vi "AlliGator All ROIs Decay Fit Non-Interactive (Fast + Individual IRF) v2.vi"(8 "error in (no error)":errorcluster, 11 "AlliGator Internal Variables DVR":refnum<data-value>) -> (0 "error out":errorcluster, 1 "Message":string, 3 "AlliGator Internal Variables DVR":refnum<data-value>)   [LabVIEW 2021, in "AlliGator Decay Analysis.lvlib" / "AlliGator Decay Fit.lvlib"]
doc: "Performs multi-ROIs NLSF decay fits for the selected ROIs.\n\nEach ROI has its own associated IRF."
uses:
  AlliGator Decay Fit.lvlib
  AlliGator Variables List.ctl
  AlliGator Globals, Variables & Constants.lvlib
  Image/Named ROI Description.ctl
  Image/Image.lvlib
  AlliGator Decay Processing.lvlib
  AlliGator Source Image.lvlib
  <vilib>/vision/Image Controls.llb/IMAQ Image.ctl
  Strings/Strings.lvlib
  Time/Time.lvlib
  AlliGator Settings.lvlib
  AlliGator Settings List.ctl
  AlliGator Abort.vi
  Variant/Variant to Data/Variant to Data.lvlib
  GUI/GUI.lvlib
  AlliGator Decay Preprocessing.lvlib
  Arrays/Arrays.lvlib
  Fits/Fits.lvlib
  <vilib>/ErrorRing/Error Ring.xnode
  <vilib>/Utility/error.llb/Error Cluster From Error Code.vi
  Notebook/Notebook.lvlib
  Rich Text Box/Rich Text Box.lvlib
  Sound/Sound.lvlib
  Graphs/XY Graph/XY Graph Selected Plot Info+Flag.ctl
  Graphs/XY Graph/XY Graph Add-Ons.lvlib
  <vilib>/Utility/miscctls.llb/LVPoint32TypeDef.ctl
  Graphs/XY Graph/XY Graph Refnum.ctl
  AlliGator Decay Fit Parameter Map.lvlib
  Variant/Variant to Data/Variant to U16.vi
  Variant/Variant to Data/Variant to Boolean.vi
  Phasor/Phasor Reference Series.ctl
  Phasor/Phasor.lvlib
  Phasor/Phasor (g, s).ctl
  Phasor/Calibration Phasor (m, phi).ctl
  AlliGator Data Series Type.ctl
  AlliGator Files.lvlib
  AlliGator Internal Variables v2.ctl
  AlliGator Internal Variables.lvlib
  AlliGator Decay Metadata v3.ctl
  AlliGator Phasor Graph.lvlib
  AlliGator Raw Phasor Plot Data v4.ctl
  AlliGator Baseline Subtraction Method.ctl
  AlliGator Decay Background Subtraction Info.ctl
  Graphs/XY Graph/XY Graph Plot Shift Method.ctl
  Graphs/XY Graph/XY Graph Plot Shift Parameters.ctl
  AlliGator Decay Extrapolation Parameters.ctl
  AlliGator FLI Dataset Type.ctl
  Phasor/Phasor Harmonic Data.ctl
  AlliGator Phasor Multi-Harmonic Data.ctl
  AlliGator Phasor Plot.lvlib
  AlliGator Displayed Image.ctl
  Fits/IRF(X)PSED/Decay Fit Parameters & Derived Quantities List.ctl
  Fits/IRF(X)PSED/Decay Fit Parameters In List.ctl
  AlliGator Decay Fit Parameter Constraints 2.ctl
  Fits/Decay Convolution/Decay Model.ctl
  Fits/Residual Type.ctl
  Fits/Fit Calculation Method.ctl
  Fits/Non-linear Fitting Algorithm.ctl
  AlliGator Decay Fit Options & Parameters v2.ctl
  Fits/IRF(X)PSED/Fit Weights Type.ctl
  AlliGator Gate Image Set.ctl
  AlliGator Gate Arithmetic.ctl
  AlliGator Dataset Channel.ctl
  AlliGator Dual-Channel Datasets.lvlib
  AlliGator Decay Preprocessing Parameters.ctl
  Phasor/Phasor Standard Deviation Options.ctl
  Phasor/Phasor Calibration Map v2.ctl
  Fits/Non-linear Fitting Method v2.ctl
  Fits/IRF(X)PSED/Decay Fit Options v2.ctl
  Fits/IRF(X)PSED/MLE Baseline Offset Type.ctl
  AlliGator Parameter Maps Data.ctl
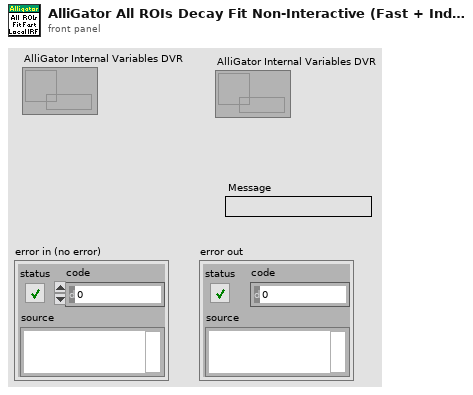
[diagram p1: front panel]
types:
  T1 = typedef "AlliGator Globals, Variables & Constants.lvlib/AlliGator Variables List.ctl" = enum16{"---- GUI ----", "GUI:Initialization Status", "GUI:State Indicators Refnum", "GUI:Original AlliGator Menu Items", "GUI:Current Action Loop State", "GUI:Script in progress", "GUI:Playback", "GUI:Loop Playback", "GUI:Search ROI Used", "GUI:Search ROI", "Decay Graph Max Legend Size", "Intensity Graph Max Legend Size", "Decay Statistics Graph Max Legend Size", "Phasor Graph Max Legend Size", "Phasor Ratio Graph Max Legend Size", "Lifetime Graph Max Legend Size", "---- Files ----", "Files:Export Dataset Frames as Individual Files", "Files:Show Batch Export Help Balloons", "Files:Frames in Dataset", "Files:ptu File Frame Start Indices", "Files:Current Frame in Dataset", "Files:Current Frame Timestamp", "Files:Dataset Loaded", "Files:Dataset Metadata", "Files:Dataset Channel", "Files:Dataset Data Description", "Files:Background Dataset Metadata", "Files:Background Dataset Channel", "Files:Background Dataset Data Description", "Files:Background File Subtraction", "Files:Background File Path", "Files:Background File Pile-up Correction", "Files:Background File Pixel Well Capacity", "Files:Background File Scaling Factor", "Files:Current Dataset Load Settings", "Files:Dataset Path", "Files:ICCD-specific Information", "Files:Macrotime Gate Separation", "------ Python Plugins ------", "Python Plugins:Information", "Python Plugins:Python Session", "Python Plugins:Valid Python Session?", "---- Source Image ----", "Source Image:ROIs", "Source Image:Current ROI", "Source Image:ROI Event Refnum", "X_Source Image Display Range", "X_Source Image Palette Information", "X_Type of Displayed Image", "X_Time Gate Slider", "Source Image:Palette List", "Source Image:Scale", "Source Image:ROI Overlay Color", "Source Image:Overlay to Erase", "Source Image:Is Displayed Image Accumulated", "Source Image:White Light Image Modified", "Source Image:Mask Image Modified", "---- Image Profile Window ----", "Image Profile:Overlay ROI in Source Image", "Image Profile:Window Event Refnum", "Image Profile:IntensityType", "Image Profile:Intensity Average Type", "Image Profile:Intensity-weighted SDV", "Image Profile:Box Profile Type", "Image Profile:Window Open", "Image Profile:Plotted Fit Parameter", "------ Phasor Graph -------", "Phasor Graph:Show Line", "---- Phasor Plot ---", "Phasor Plot:Parameters Changed", "Phasor Plot:FLI Dataset Modified since last Calculation", "Phasor Harmonics Data", "Selected Phasor Harmonics", "Phasor Harmonic Manager Event Refnum", "Phasor Plot:ROIs", "Phasor Plot:Current ROI", "Phasor Plot:ROI Event Refnum", "Phasor Plot:Image Reference Points", "Phasor Plot:Computed", "Phasor Plot:Palette Information", "Phasor Plot:Palette List", "Phasor Plot:Phasor Ratio Palette Information", "Phasor Plot:Phasor Ratio Palette List", "Phasor Plot:Image Scale", "Phasor Plot:Image Overlay to Erase", "Phasor Plot:Image Elements to Update", "Phasor Plot:Current Calculation Parameters", "Phasor Plot:Current Calibration Options", "Phasor Plot:Reset Cumulated Phasor Plot", "Phasor Plot:Reference 1", "Phasor Plot:Lifetime Reference 1", "Phasor Plot:Reference 1 Frequency", "Phasor Plot:Reference 2", "Phasor Plot:Lifetime Reference 2", "Phasor Plot:Reference 2 Frequency", "---- Decay Analysis ----", "Number of Selected Decays to Fit", "LS Fit Results", "LAR Fit Results", "BS Fit Results", "Last Decay Max - Min", "Best Fit Parameters", "Best Fit Parameter Names", "Actual Size X", "Actual Size Y", "Binning X", "Binning Y", "Actual # Gates", "Dataset Number", "Gates to...", "Gates Skipped", "Gates to keep", "Gate Step", "Gate Separation", "Reversed Gates", "Pile-up Correction", "Pixel Well Capacity", "Background Subtracted", "Background Subtraction Method", "Background Definition Range", "Background File (deprecated)", "Number of Dataset Accumulated", "Array of Accumulated Dataset Paths", "Do Averaged Datasets", "Destination File Path", "Process Plot Target", "Use 1/D as Phasor Frequency", "---- Decay Fit Parameter Map -----", "Decay Fit Parameter Map:Palette Information", "Decay Fit Parameter Map:Palette List", "------- Local Decay Window ---------", "Local Decay Graph Window:Event Refnum", "Local Decay Graph Window:Use normalized IRF for convolution", "----- Miscellaneous ----", "Misc:Skippable Dialog Windows Status"}
  T2 = typedef "IMAQ Image.ctl" = refnum<image>
  T3 = typedef "AlliGator Settings.lvlib/AlliGator Settings List.ctl" = enum16{"GUI:Visible Settings Tab", "GUI:Last Run Version", "Source Image:Use Image Histogram for Contrast", "Source Image:Low Count Pixels Rejection Options", "Source Image:High Count Pixels Rejection Options", "Source Image:Use Image Brightness", "Source Image:Blend Overlay with Image Background", "Source Image:Use Fixed ROI Diameter", "Source Image:ROI Diameter", "Source Image:ROI Center Color", "Source Image:Peak Threshold", "Source Image:Intensity Threshold", "Source Image:Image Binning Options", "Source Image:Image Smoothing Options", "Source Image:Image Histogram Active", "Source Image:Invert Binary Mask", "Source Image:Hot Pixel Removal", "Source Image:Overlay Analyzed ROI Center", "Source Image:Auto-Adjust Contrast", "Source Image:Histogram Lower Percentile", "Source Image:Histogram Upper Percentile", "Source Image:Save Source Image", "Source Image:Scale Bar Options", "Source Image:Image Resolution (Pixel Size)", "Source Image:Flatfield Correction", "Source Image:Show Dead Left Columns Correction", "Source Image:Dead Left Columns Correction", "Source Image:Image Pre-Processing Operations Order", "Data Information:Gate Width", "Data Information:Nanotime Gate Separation", "Data Information:Macrotime Gate Separation", "Data Information:Gate Step", "Data Information:# Gates", "Data Information:Gate Image Exposure", "Data Information:Gate Image Integration", "Data Information:Gates to Skip", "Data Information:Gates to Keep", "Data Information:Define Gates to", "Data Information:Channel Name", "Data Information:Available Channel Names", "Data Information:Channel Arithmetic", "Data Information:Background File Subtraction", "Data Information:Background File", "Data Information:Background Scaling Factor", "Data Information:Background Pile-up Correction", "Data Information:Background Pixel Well Capacity", "Data Information:Laser Period", "Data Information:SYNC Period", "Data Information:Pile-up Correction", "Data Information:Pixel Well Capacity", "Data Information:Dataset Scaling Factor", "Fluorescence Decay_Decay Pre-Processing:Reverse Gates", "Fluorescence Decay_Decay Pre-Processing:Verbose Decay Pre-Processing", "Fluorescence Decay_Decay Pre-Processing:Use Decay Pre-Processing", "Fluorescence Decay_Decay Pre-Processing:Background Subtraction", "Fluorescence Decay_Decay Pre-Processing:Background Definition Range", "Fluorescence Decay_Decay Pre-Processing:Baseline Subtraction Method", "Fluorescence Decay_Decay Pre-Processing:Decay Pre-Processing Operations Order", "Fluorescence Decay_Decay Pre-Processing:Smoothing Parameter", "Fluorescence Decay_Decay Pre-Processing:Shift Decay", "Fluorescence Decay_Decay Pre-Processing:Decay Shift Parameters", "Fluorescence Decay_Decay Pre-Processing:Fold Decay", "Fluorescence Decay_Decay Pre-Processing:# Folds", "Fluorescence Decay_Decay Pre-Processing:1-Normalize Decay", "Fluorescence Decay_Decay Pre-Processing:[0-1]-Normalize Decay", "Fluorescence Decay_Decay Pre-Processing:Smoothen Decay", "Fluorescence Decay_Decay Pre-Processing:Extrapolate Decay", "Fluorescence Decay_Decay Pre-Processing:Use Periodicity", "Fluorescence Decay_Decay Pre-Processing:Use Cursors", "Fluorescence Decay_Decay Pre-Processing:Tail Fraction", "Fluorescence Decay_Decay Pre-Processing:Head Fraction", "Fluorescence Decay_Decay Pre-Processing:Additional Points", "Fluorescence Decay_Decay Pre-Processing:Straighten Decay", "Fluorescence Decay_Decay Pre-Processing:Constant Background", "Fluorescence Decay_Decay Pre-Processing:Pixel-Normalize Decay", "Fluorescence Decay_Advanced Analysis:Extract IRF instead of Decay", "Fluorescence Decay_Advanced Analysis:IRF Extraction Options", "Fluorescence Decay_Advanced Analysis:IRF Optimization Options", "Fluorescence Decay_Advanced Analysis:Square Pulse Options", "Fluorescence Decay_Advanced Analysis:IRF Order", "Fluorescence Decay_Advanced Analysis:IRF Time Constants", "Fluorescence Decay_Advanced Analysis:Wavelet Analysis Options", "Fluorescence Decay_Advanced Analysis:Average Lifetime Options", "Fluorescence Decay_Fit Options:Fit Options", "Fluorescence Decay_Fit Options:Use Legacy Fitting Approach", "Fluorescence Decay_Fit Options:Use Data Information Laser Period", "Fluorescence Decay_Fit Parameters:Displayed Fit Parameters", "Fluorescence Decay_Fit Parameters:Fit Parameter Constraints", "Fluorescence Decay_Fit Parameters:Export Tabulated Results", "Fluorescence Decay_Fit Parameters:MLE Baseline Offset Type", "Fluorescence Decay_Fit Parameters:MLE Baseline Offset", "Fluorescence Decay_Fit Parameters:Guess Parameter Names", "Fluorescence Decay_Fit Parameters:Guess Parameter Values", "Fluorescence Decay_Fit Parameters:Guess Parameters Options", "Fluorescence Decay_Styles:Show Last Decay Only", "Fluorescence Decay_Styles:Decay Graph Color Array", "Fluorescence Decay:Decay Graph Active", "Fluorescence Decay Statistics:Min Peak Value", "Fluorescence Decay Statistics:Reject Low Decay Peak Pixels", "Fluorescence Decay Statistics:Reject High Decay Peak Pixels", "Fluorescence Decay Statistics:Max Peak Value", "Time Traces:Use File Timestamp", "Time Traces:Time Step", "Time Traces:Use Intensity Correction File", "Time Traces:Intensity Correction File", "Phasor Plot:Phasor Plot Smoothing Options", "Phasor Plot:Phasor Plot Size", "Phasor Plot:Phasor Plot Graphics Options", "Phasor Plot:Cumulative Phasor Plot", "Phasor Plot:Use Phasor Brightness", "Phasor Plot:Blend Overlay with Phasor Background", "Phasor Plot:Save Phasor Plot", "Phasor Plot:Show References", "Phasor Plot:Phasor Ratio Decay Range", "Phasor Plot:Exponential Fading", "Phasor Plot:Phasor Ratio Reference Colors", "Phasor Plot:Reference Radius", "Phasor Plot:Show Color Map Vertices", "Phasor Plot:Phasor Plot Active", "Phasor Plot:Phasor Ratio Color Map Type", "Phasor Plot:Phasor Ratio Color Map", "Phasor Plot:Phasor Ratio Display Range", "Phasor Plot:Selected Image ROI(s)", "Phasor Plot:All Image ROIs", "Phasor Plot:Selected Phasor Plot ROI(s)", "Phasor Plot:All Phasor Plot ROIs", "Phasor Plot:Phasor Ratio Color-Coded Quantity", "Phasor Plot:Store Phasor Harmonics", "Phasor Plot:Draw Reference Segment", "Phasor Plot:User-Defined Quantity", "Phasor Graph:Phasor Frequency", "Phasor Graph:Phasor Ratio Type", "Phasor Graph:Pixel-level Phasor Computation", "Phasor Graph:Save Phasor Graph", "Phasor Graph:Phasor Graph Active", "Phasor Graph:Phasor SDV Options", "Phasor Calibration:Use Backup Calibration if needed", "Phasor Graph:Define Shortest Lifetime as", "Phasor Calibration:Backup Calibration Type", "Phasor Calibration:Calibration Type", "Phasor Calibration:Calibration Lifetime", "Phasor Calibration:Calibration Map Algorithm", "Single-Exponential Phasor Locus (SEPL):Gate Parameters", "Single-Exponential Phasor Locus (SEPL):User-defined Gate", "Single-Exponential Phasor Locus (SEPL):User-defined IRF", "Single-Exponential Phasor Locus (SEPL):Phasor Parameters", "Single-Exponential Phasor Locus (SEPL):Decay & IRF Parameters", "Single-Exponential Phasor Locus (SEPL):Display Parameters", "Lifetime Analysis:Decay Analysis Parameters", "Lifetime Analysis:Lifetime Map Active", "Plugins:Python Settings", "Miscellaneous:Verbose Mode", "Miscellaneous:Beep after Script", "Miscellaneous:Saved Image File Format", "Miscellaneous:Exported Gate Image Settings", "Miscellaneous:Include Loading in Timing", "Miscellaneous:Verbose Settings Mode", "Miscellaneous:Histogram Options", "Miscellaneous:Beep on Error", "Miscellaneous:# Logical Processors Used", "Miscellaneous:ROI Description Max Characters", "Miscellaneous:Verbose Error Mode", "Miscellaneous:Transparent Mask Color"}
  T4 = typedef "Image.lvlib/Named ROI Description.ctl" = cluster{"ROI Descriptor":T5, "ROI Name":string, "Overlay Color":u32}
  T5 = typedef "ROI Descriptor" = cluster{"Global Rectangle":i32[], "Contours":cluster{"ID":enum32{"External", "Internal"}, "Type":u32, "Coordinates":i32[]}[]}
  T6 = typedef "AlliGator Internal Variables.lvlib/AlliGator Internal Variables v2.ctl" = cluster{"Displayed Image":T2, "White Light Image":T2, "Mask Image":T2, "ROI Mask Image":T2, "Current Dataset Images 1":T7, "Background Dataset Images 1":T7, "Current Dataset Images 2":T7, "Background Dataset Images 2":T7, "Current Dataset Arithmetic Images":T7, "Accumulated Dataset Images 1":T7, "Accumulated Dataset Images 2":T7, "Accumulated Dataset Arithmetic Images":T7, "Phasor Plot Image":T2, "Decay Fit Parameter Map Image":T2, "Single Data Point Path":path, "White Light Image Path":path, "Mask Image Path":path, "Time-Series Folder":path, "[Time-Series Paths]":path[], "Current Dataset":i32, "Single Dataset Type":T8, "Current Folder":string, "AlliGator Data Series Type":T9, "# Datasets":i32, "Dual-Channel Dataset":bool, "Selected Channel Name":string, "Dataset Channel":T10, "Channel Arithmetic":T11, "Dual-Channel Background Dataset":bool, "Background Channel":T10, "Dual-Channel Accumulated Dataset":bool, "Start Time":dbl, "[Time-Series Timestamps]":dbl[], "[Intensity Corrections]":dbl[], "Time Series Script":bool, "Type of Displayed Image":T12, "Gate Image Slide":u16, "# Gates":i32, "ROIs":T4[], "ROI Decay":cluster{"t Array":dbl[], "I Array":dbl[]}, "Valid Decay":bool, "Decay  Metadata":T13, "Reference Decay Plot Name":string, "Reference Decay":cluster{"t Array":dbl[], "I Array":dbl[]}, "Decay Shift Plot":cluster{"Time Stamps":dbl[], "Decay Shifts":dbl[]}, "[Decays Max Values]":sgl[], "[Decays Min Values]":sgl[], "Calibration Phasor":T19, "Calibration Phasor Series":T20, "Phasor Calibration Map":T21, "Calibration Map MD5 Digest":string, "Last Raw Phasor":T22, "Last Calibrated Phasor":T22, "Last Calibrated Phasor SDV":T22, "Phasor Graph:Phasor Plot":cluster{"g Array":dbl[], "s Array":dbl[]}, "Phasor Graph:Phasor SDV Plot":cluster{"g Array":dbl[], "s Array":dbl[]}, "[Phasor Graph:Raw Phasor Plots]":T23[], "Phasor Plot locked to Ref 1":i32, "[Phasor Plot(s) locked to Ref 1]":i32[], "[Phasor Plot(s) locked to Ref 2]":i32[], "[Pixel Phasors]":T22[], "[[Sum Image]]":dbl[][], "[[CSG Phasors]]":csg[][], "[[Valid Pixel?]]":bool[][], "I/m/phi Dataset":cluster{"I/m/phi Dataset?":bool, "Base Frequency":dbl[unit], "Harmonic Orders":u8[]}, "Multi Phasor Plot Data":T25, "Decay Fit Options & Parameters":T27, "Fit Options: Decay Preprocessing Parameters":T38, "Fit Options: Reference Decay":cluster{"t Array":dbl[], "I Array":dbl[]}, "Is Full Image Parameters Map":bool, "Is Single-Pixels Parameters Map":bool, "NLSF Parameters Map X Resolution":i32, "NLSF Parameters Map Y Resolution":i32, "[Single Decay Fit Parameters]":dbl[], "Fit Model":T29, "[[Multiple Decays Fit Parameters]]":dbl[][], "[[Multiple Decays Fit Parameter SDVs]]":dbl[][], "[[IRFs]]":dbl[][], "IRF Array Time Axis":dbl[], "Decay Array Time Axis":dbl[], "[Decay Fit Parameter Names]":T39[], "[[Phasor Ratios]]":dbl[][], "[[Average Lifetimes]]":dbl[][], "Amplitude Weighted Average Lifetime":bool, "[Decay Sum]":dbl[], "Parameter Maps":T40[], "[[User-defined Quantities]]":dbl[][], "User-defined Quantity":string}
  T7 = typedef "AlliGator Internal Variables.lvlib/AlliGator Gate Image Set.ctl" = cluster{"SGL Image Max":T2, "SGL Image Sum":T2, "SGL Gate Images":T2[], "SGL Image Min":T2}
  T8 = typedef "AlliGator Files.lvlib/AlliGator FLI Dataset Type.ctl" = enum16{"HDF5 FLI Dataset", "Gate Image Folder", ".sdt FLI Dataset (Becker & Hickl)", ".ptu FLI Dataset (PicoQuant)", "SS1 FLI Dataset", "SS2 FLI Dataset", "I/m/phi Dataset", ".bin FLI Dataset (PicoQuant Binned)", ".bin FLI Dataset (Piccolo Binned)"}
  T9 = typedef "AlliGator Files.lvlib/AlliGator Data Series Type.ctl" = enum16{"Not a Supported Series", "Gate Images Folder Series", "SwissSPAD 2 Dataset Series", "B&H FLI Dataset Series", "PicoQuant PTU FLI Dataset Series", "PicoQuant BIN FLI Dataset Series", "Piccolo hist BIN FLI Dataset Series", "HDF5 FLI Dataset Series"}
  T10 = typedef "AlliGator Dual-Channel Datasets.lvlib/AlliGator Dataset Channel.ctl" = enum16{"G2", "INT"}
  T11 = typedef "AlliGator Settings.lvlib/AlliGator Gate Arithmetic.ctl" = enum16{"None", "INT-G2", "G2/INT*<INT>", "(1 - G2/INT)*<INT>"}
  T12 = typedef "AlliGator Source Image.lvlib/AlliGator Displayed Image.ctl" = enum16{"Single Gate", "Sum of All Gates", "Max of All Gates", "Min of All Gates", "-", "White Ligth Image", "Mask Image"}
  T13 = typedef "AlliGator Phasor Graph.lvlib/AlliGator Decay Metadata v3.ctl" = cluster{"ROI Descriptor":T5, "ROI Center":cluster{"X":i32, "Y":i32}, "Decay Background Subtraction Info":T14, "Decay Reverted":bool, "Decay Smoothened":bool, "Decay Straightened":bool, "Fitted Tau (Decay Straightening)":dbl, "Decay Shift Parameters":T16, "Decay Shifted":bool, "Decay Extrapolated":bool, "Decay Extrapolation Parameters":T18, "Decay Normalized":bool, "Fold Decay":bool, "# Folds":u32}
  T14 = typedef "AlliGator Decay Analysis.lvlib/AlliGator Decay Preprocessing.lvlib/AlliGator Decay Background Subtraction Info.ctl" = cluster{"Laser Period":dbl[unit], "Gate Duration":dbl[unit], "Baseline Subtraction Method":T15, "Background Definition Range":cluster{"Min Gate":dbl[unit], "Max Gate":dbl[unit]}, "Total Intensity w/o Bkgd Subtraction":dbl, "Bkgd-subtracted Intensity (exp)":dbl, "# Data Points":i32, "Background/Gate":dbl, "Fitted Lifetime":dbl[unit], "Bkgd-subtracted Intensity (theo)":dbl}
  T15 = typedef "AlliGator Decay Analysis.lvlib/AlliGator Decay Preprocessing.lvlib/AlliGator Baseline Subtraction Method.ctl" = enum16{"Mean", "Min", "Square Gated Single-Exponential", "File", "Constant"}
  T16 = typedef "XY Graph Add-Ons.lvlib/XY Graph Plot Shift Parameters.ctl" = cluster{"Type":T17, "Shift":dbl[unit], "Threshold":dbl, "Rotate":bool}
  T17 = typedef "XY Graph Add-Ons.lvlib/XY Graph Plot Shift Method.ctl" = enum16{"Default", "CFD", "Threshold", "Cross-Correlation"}
  T18 = typedef "AlliGator Decay Analysis.lvlib/AlliGator Decay Preprocessing.lvlib/AlliGator Decay Extrapolation Parameters.ctl" = cluster{"Additional Points":u32, "Head Fraction":dbl, "Fitted Tau":dbl, "Use Periodicity":bool, "Use Cursors":bool, "Tail Fraction":dbl}
  T19 = typedef "Phasor.lvlib/Calibration Phasor (m, phi).ctl" = cluster{"m":dbl, "phi":dbl, "Phasor Frequency":dbl[unit], "Reference Lifetime":dbl[unit]}
  T20 = typedef "Phasor.lvlib/Phasor Reference Series.ctl" = cluster{"m Array":dbl[], "phi Array":dbl[], "Phasor Frequency":dbl[unit], "Calibration Lifetime":dbl[unit]}
  T21 = typedef "Phasor.lvlib/Phasor Calibration Map v2.ctl" = cluster{"Phasor Frequency":dbl[unit], "Calibration Lifetime":dbl[unit], "ROI Centers":cluster{"X":i32, "Y":i32}[], "ROI Descriptors":T5[], "Map Resolution X":i32, "Map Resolution Y":i32, "z Array":cdb[]}
  T22 = typedef "Phasor.lvlib/Phasor (g, s).ctl" = cluster{"g":dbl, "s":dbl}
  T23 = typedef "AlliGator Phasor Graph.lvlib/AlliGator Raw Phasor Plot Data v4.ctl" = cluster{"Phasor Plot Name":string, "Raw Phasor Plot":T22[], "Phasor Frequency":dbl[unit], "[Decay Metadata]":T13[], "Raw Phasor Plot SDV":T22[], "Phasor SDV Options":T24, "[Calibration Phasor]":T19[]}
  T24 = typedef "Phasor.lvlib/Phasor Standard Deviation Options.ctl" = cluster{"Compute Estimated SDV":bool, "# Replicas":u32, "Use Estimated Average Phasor":bool}
  T25 = typedef "AlliGator Phasor Plot.lvlib/AlliGator Phasor Multi-Harmonic Data.ctl" = cluster{"Base Frequency":dbl[unit], "# Harmonics":u8, "Harmonic Orders":u8[], "Phasor Plot Settings Checksum":u64, "Phasor Harmonic Data Array":T26[]}
  T26 = typedef "Phasor.lvlib/Phasor Harmonic Data.ctl" = cluster{"Phasor Harmonic Name":string, "Phasor Plot Settings Checksum":u64, "Phasor Frequency":dbl[unit], "Base Frequency":dbl[unit], "Harmonic Order":u8, "Phasor Plot Parameters":string, "Phasor Array [[CSG]]":csg[][], "Dataset File Path":path}
  T27 = typedef "AlliGator Decay Fit Parameter Map.lvlib/AlliGator Decay Fit Options & Parameters v2.ctl" = cluster{"SYNC Period":dbl[unit], "Fit Options":T28, "Fit Parameter Constraints":T35[], "MLE Baseline Offset":dbl, "MLE Baseline Offset Type":T37}
  T28 = typedef "Fits.lvlib/Decay Fit Options v2.ctl" = cluster{"Show Fit Residuals":bool, "Fit Model":T29, "Residual Type":T30, "Max Decay Percentile":dbl, "Min Decay Percentile":dbl, "Show Full Decay":bool, "Weights":T31, "Fitting Method":T32, "Compute Parameter Uncertainties":bool, "Periodic Boundaries":bool, "Model Calculation":T33, "Period":dbl[unit], "Termination Criteria":cluster{"Max Iterations":i32, "Max Function Calls":i32, "Max Time":dbl[unit], "Function Tolerance":dbl, "Parameter Tolerance":dbl, "Gradient Tolerance":dbl, "Min Lambda":dbl, "Max Lambda":dbl, "Initial Tick Count":u32}, "Offset Resolution":dbl[unit], "Use Local IRF":bool, "Fitting Algorithm":T34}
  T29 = typedef "Fits.lvlib/Decay Model.ctl" = enum16{"1-Exponential", "2-Exponentials"}
  T30 = typedef "Fits.lvlib/Residual Type.ctl" = enum16{"Standard", "Normalized", "Reduced"}
  T31 = typedef "Fits.lvlib/Fit Weights Type.ctl" = enum16{"Unweighted", "1/Variance", "Best of All"}
  T32 = typedef "Fits.lvlib/Non-linear Fitting Method v2.ctl" = enum16{"Least Square", "Least Absolute Residual", "Bisquare", "MLE", "-", "Best of All"}
  T33 = typedef "Fits.lvlib/Fit Calculation Method.ctl" = enum16{"Simulation", "Convolution", "Integration"}
  T34 = typedef "Fits.lvlib/Non-linear Fitting Algorithm.ctl" = enum16{"Levenberg-Marquardt", "Trust-Region Dogleg"}
  T35 = typedef "AlliGator Decay Analysis.lvlib/AlliGator Decay Fit.lvlib/AlliGator Decay Fit Parameter Constraints 2.ctl" = cluster{"Fit Parameter":T36, "Min Value":dbl, "Max Value":dbl, "Global":bool, "Used":bool}
  T36 = typedef "Fits.lvlib/Decay Fit Parameters In List.ctl" = enum16{"Offset", "Baseline", "A_1", "tau_1", "A_2", "tau_2"}
  T37 = typedef "Fits.lvlib/MLE Baseline Offset Type.ctl" = enum32{"Absolute", "Percentage"}
  T38 = typedef "AlliGator Decay Analysis.lvlib/AlliGator Decay Preprocessing.lvlib/AlliGator Decay Preprocessing Parameters.ctl" = cluster{"Background Subtraction":bool, "Straighten Decay":bool, "Reverse Gates":bool, "1-Normalized Decay":bool, "Smoothen Decay":bool, "Smoothing Parameter":dbl, "Shift Decay":bool, "Decay Shift Parameters":T16, "Extrapolate Decay":bool, "Additional Points":u32, "Head Fraction":dbl, "Pixel-Normalize Decay":bool, "Use Periodicity":bool, "Use Cursors":bool, "Tail Fraction":dbl, "Use Decay Pre-Processing":bool, "Fold Decay":bool, "# Folds":u32, "[0-1]-Normalized Decay":bool}
  T39 = typedef "Fits.lvlib/Decay Fit Parameters & Derived Quantities List.ctl" = enum16{"Offset", "Baseline", "A_1", "tau_1", "A_2", "tau_2", "<tau>_a", "f1_a", "f2_a", "<tau>_i", "f1_i", "f2_i", "-", "R^2", "Chi^2"}
  T40 = typedef "AlliGator Parameter Maps Data.ctl" = cluster{"Map Set Name":string, "[Parameter Names]":string[], "[[Parameters]]":dbl[][], "[[Parameter SDVs]]":dbl[][], "Decay Array Time Axis":dbl[], "[[IRFs]]":dbl[][], "IRF Array Time Axis":dbl[]}
  T41 = typedef "AlliGator Settings.lvlib/AlliGator Pixel Counts Constraints.ctl" = cluster{"High Count Pixels Rejection Options":T42, "Low Count Pixels Rejection Options":T43}
  T42 = typedef "AlliGator Settings.lvlib/AlliGator High Count Pixels Rejection Options.ctl" = cluster{"Background High Threshold Factor":dbl, "Fixed High Background Threshold":dbl, "Reject High Count Pixels":bool, "High Percentile":dbl}
  T43 = typedef "AlliGator Settings.lvlib/AlliGator Low Count Pixels Rejection Options.ctl" = cluster{"Background Low Threshold Factor":dbl, "Fixed Low Background Threshold":dbl, "Reject Low Count Pixels":bool, "Low Percentile":dbl}
  T44 = cluster{"Decay Peak Constraint":bool, "Min":dbl, "Max":dbl}
  T45 = typedef "XY Graph Add-Ons.lvlib/XY Graph Selected Plot Info+Flag.ctl" = cluster{"Multiplot XY Graph":T46, "Mouse Coordinates":T47, "Plot Index":i32, "Flag":bool}
  T46 = typedef "XY Graph Add-Ons.lvlib/XY Graph Refnum.ctl" = refnum<vi>
  T47 = typedef "LVPoint32TypeDef.ctl" = cluster{"Horizontal":i32, "Vertical":i32}
  T48 = cluster{"t Axis":dbl[], "ROI Intensity Array":dbl[]}
  T49 = cluster{"IRF Array Time Axis":dbl[], "[IRF Values]":dbl[]}
  T50 = typedef "Rich Text Box.lvlib/Text Formatting.ctl" = cluster{"Font":string, "Text Color":T51, "Text Background Color":T51, "Text Style":enum16{"Regular", "Bold", "Italic", "Underline", "Strikeout"}, "Font Size (Points)":dbl, "Text Alignment":i32}
  T51 = typedef "Rich Text Box.lvlib/Text Colors.ctl" = enum16{"Unchanged", "Black", "Blue", "Brown", "Gray", "Green", "Orange", "Pink", "Red", "White"}
  T52 = typedef "AlliGator Decay Analysis.lvlib/AlliGator Decay Fit.lvlib/AlliGator Decay Fit Output Options.ctl" = cluster{"Fit Model":T29, "Decay Fit Parameter Array":T39[]}
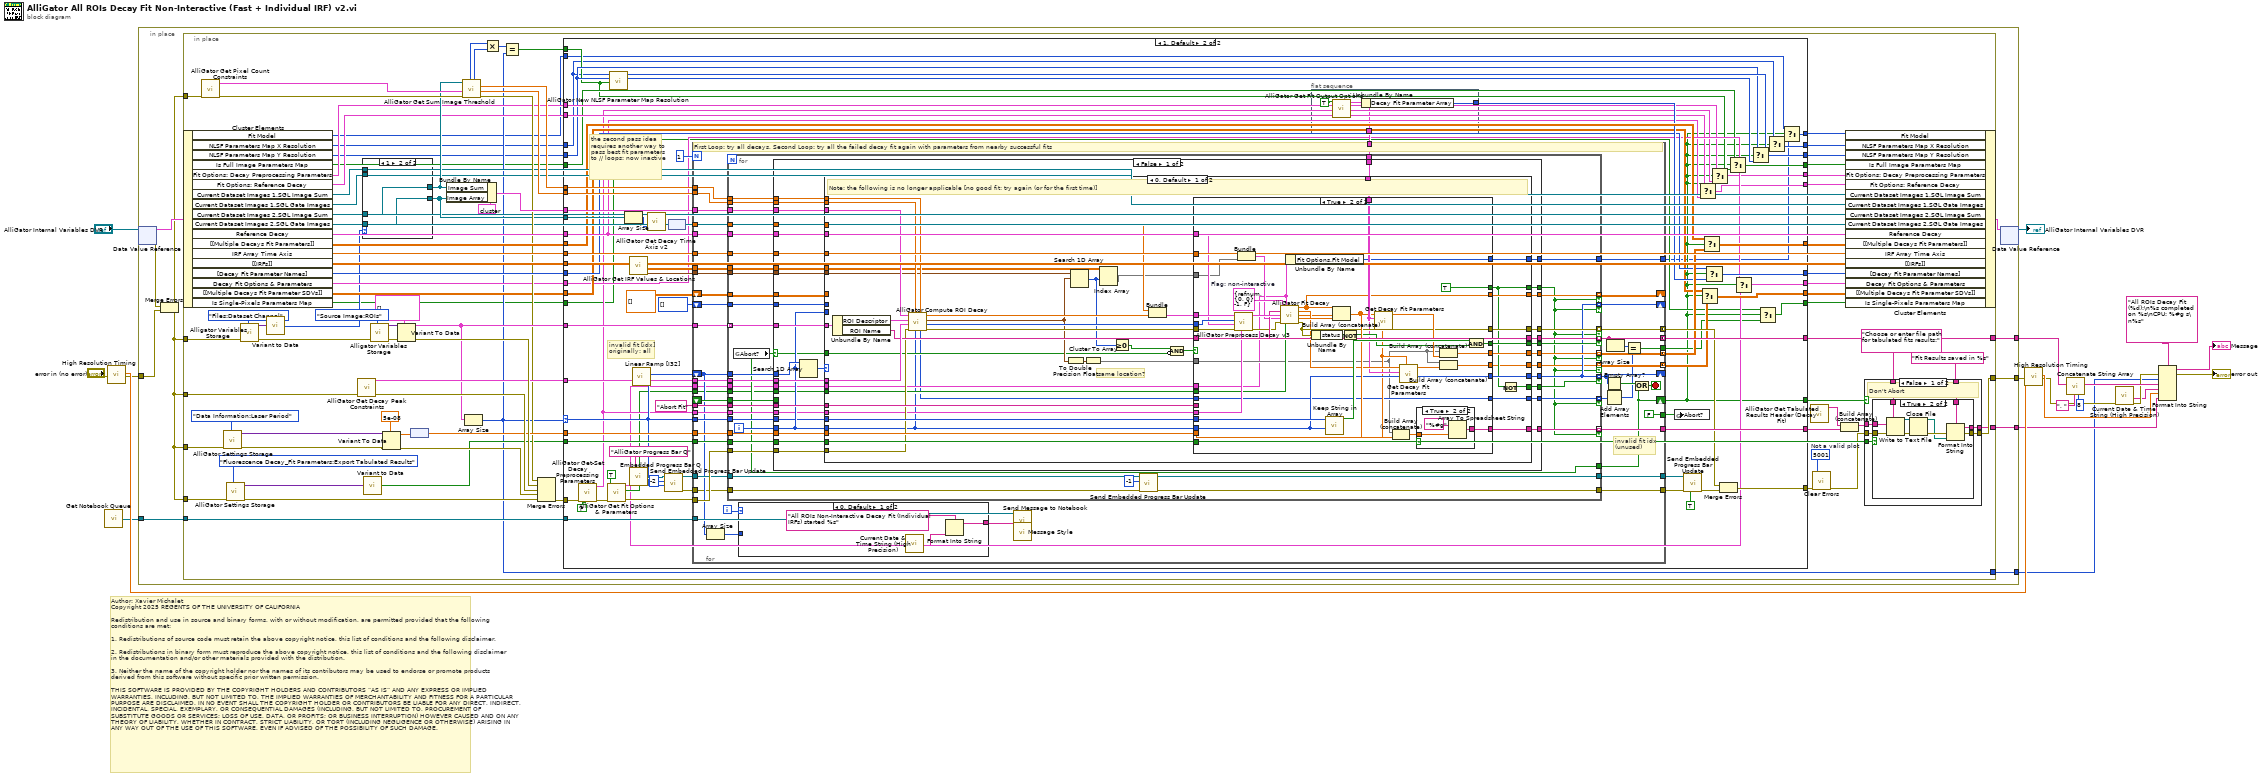
[diagram p0: block diagram]
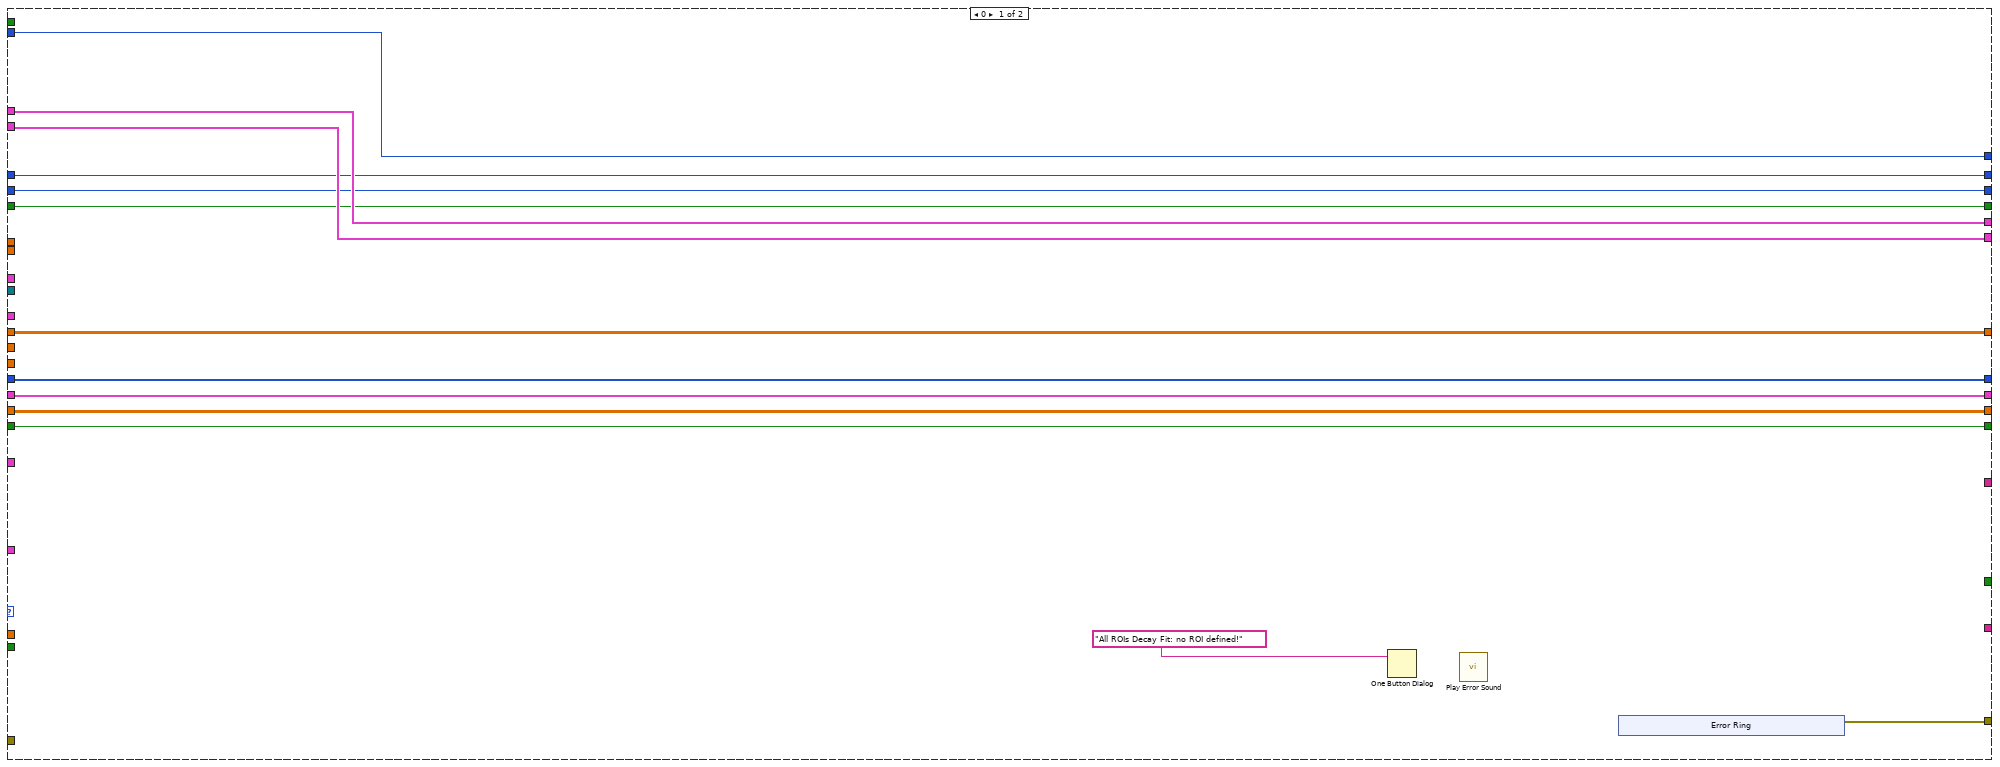
[diagram p3: hidden frame]
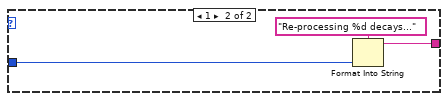
[diagram p4: hidden frame]
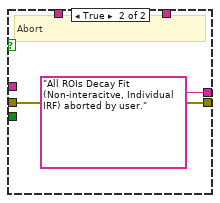
[diagram p10: hidden frame]
diagram:
  # "Author: Xavier Michalet\nCopyright 2025 REGENTS OF THE UNIVERSITY OF CALIFORNIA\n\nRedistribution and use in source and binary forms, with or without modification, are permitted provided that the following conditions are met:\n\n1. Redistributions of source code must retain the above copyright notice, this list of conditions and the following disclaimer.\n\n2. Redistributions in binary form must reproduce the above copyright notice, this list of conditions and the following disclaimer in the documentation and/or other materials provided with the distribution.\n\n3. Neither the name of the copyright holder nor the names of its contributors may be used to endorse or promote products derived from this software without specific prior written permission.\n\nTHIS SOFTWARE IS PROVIDED BY THE COPYRIGHT HOLDERS AND CONTRIBUTORS “AS IS” AND ANY EXPRESS OR IMPLIED WARRANTIES, INCLUDING, BUT NOT LIMITED TO, THE IMPLIED WARRANTIES OF MERCHANTABILITY AND FITNESS FOR A PARTICULAR PURPOSE ARE DISCLAIMED. IN NO EVENT SHALL THE COPYRIGHT HOLDER OR CONTRIBUTORS BE LIABLE FOR ANY DIRECT, INDIRECT, INCIDENTAL, SPECIAL, EXEMPLARY, OR CONSEQUENTIAL DAMAGES (INCLUDING, BUT NOT LIMITED TO, PROCUREMENT OF SUBSTITUTE GOODS OR SERVICES; LOSS OF USE, DATA, OR PROFITS; OR BUSINESS INTERRUPTION) HOWEVER CAUSED AND ON ANY THEORY OF LIABILITY, WHETHER IN CONTRACT, STRICT LIABILITY, OR TORT (INCLUDING NEGLIGENCE OR OTHERWISE) ARISING IN ANY WAY OUT OF THE USE OF THIS SOFTWARE, EVEN IF ADVISED OF THE POSSIBILITY OF SUCH DAMAGE."
  n1 = call "Get Notebook Queue.vi"() -> ("Notebook Queue"=w2:refnum<queue>)  [unwired: 9 in]
  n2 = call "High Resolution Timing.vi"("Error In"="error in (no error)") -> ("elapsed (relative) seconds"=w14:dbl, "Error Out"=w10:errorcluster)  [unwired: 16 in, 1 out]
  n3 = in-place {
    in-place-border: [w28] -> w9
    in-place-border: [w27] -> w11
    in-place-border: w10 -> [w24]
    in-place-border: [w25] -> w8
    in-place-border: [w23] -> w5
    in-place-border: w2 -> [w22]
    n4 = in-place-dvr #1("AlliGator Internal Variables DVR") -> (w30:T6, w26:errorcluster)
    n5 = Merge Errors(w26, w24) -> (w21:errorcluster)
    n6 = in-place {
      in-place-border: [w95] -> w28
      in-place-border: [w102] -> w27
      in-place-border: [w90] -> w25
      in-place-border: [w43] -> w23
      in-place-border: w22 -> [w67]
      in-place-border: w21 -> [w58]
      in-place-border: w21 -> [w54]
      in-place-border: w21 -> [w55]
      in-place-border: w21 -> [w56]
      in-place-border: w21 -> [w57]
      w70 = 5001  # Not a valid plot
      n7 = in-place-cluster #2(w30) -> ("Fit Model"=w32:T29, "NLSF Parameters Map X Resolution"=w38:i32, "NLSF Parameters Map Y Resolution"=w37:i32, "Is Full Image Parameters Map"=w41:bool, "Fit Options: Decay Preprocessing Parameters"=w48:T38, "Fit Options: Reference Decay"=w49:cluster{"t Array":dbl[], "I Array":dbl[]}, "Current Dataset Images 1.SGL Image Sum"=w62:T2, "Current Dataset Images 1.SGL Gate Images"=w61:T2[], "Current Dataset Images 2.SGL Image Sum"=w60:T2, "Current Dataset Images 2.SGL Gate Images"=w59:T2[], "Reference Decay"=w103:cluster{"t Array":dbl[], "I Array":dbl[]}, "[[Multiple Decays Fit Parameters]]"=w81:dbl[][], "IRF Array Time Axis"=w92:dbl[], "[[IRFs]]"=w77:dbl[][], "[Decay Fit Parameter Names]"=w76:T39[], "Decay Fit Options & Parameters"=w72:T27, "[[Multiple Decays Fit Parameter SDVs]]"=w68:dbl[][], "Is Single-Pixels Parameters Map"=w33:bool)
      n8 = call "AlliGator Get Pixel Count Constraints.vi"("error in (no error)"=w58) -> ("error out"=w110:errorcluster, "Pixel Count Constraints"=w111:T41)  [unwired: 9 in]
      n9 = call "AlliGator Settings Storage.vi"("AlliGator Settings List"=AlliGator_Settings_List."Data Information:Laser Period", "Error In"=w56) -> ("Error Out"=w85:errorcluster, "Variant Data out"=w87:variant)  [unwired: 8 in]
      n10 = call "AlliGator Settings Storage.vi"("AlliGator Settings List"=AlliGator_Settings_List."Fluorescence Decay_Fit Parameters:Export Tabulated Results", "Error In"=w57) -> ("Error Out"=w99:errorcluster, "Variant Data out"=w100:variant)  [unwired: 8 in]
      n11 = call "Alligator Variables Storage.vi"("AlliGator Variable"=AlliGator_Variables_List."Files:Dataset Channel" ("Alligator Variable"), "Error In"=w54) -> ("Error Out"=w53:errorcluster, "Data out"=w51:variant)  [unwired: 7 in, 1 out]
      n12 = call-poly "Variant to Data.vi"("Variant"=w51) -> ("U16 Value"=w50:u16)  [unwired: 8 in]
      n13 = call "AlliGator Get Decay Peak Constraints.vi"("error in (no error)"=w55) -> ("Error Out"=w106:errorcluster, "Decay Peak Constraints"=w105:T44)  [unwired: 9 in]
      n14 = case shown="1" w50 {
        tunnel: [w117 w119] -> w64
        tunnel: w62 -> [w117 _]
        tunnel: [w116 w118] -> w63
        tunnel: w61 -> [w116 _]
        tunnel: w60 -> [_ w119]
        tunnel: w59 -> [_ w118]
        frame 0, Default {
        }
        frame 1 {
        }
      }
      n15 = call-poly "Variant to Data.vi"("Variant"=w100) -> ("Value"=w74:bool)  [unwired: 8 in]
      n16 = call "Alligator Variables Storage.vi"("AlliGator Variable"=AlliGator_Variables_List."Source Image:ROIs" ("Alligator Variable"), "Error In"=w53) -> ("Error Out"=w113:errorcluster, "Data out"=w114:variant)  [unwired: 7 in, 1 out]
      n17 = Variant To Data(error in=w85, type=dbl[unit] 5e-08 ("Laser Period"), Variant=w87) -> (data=w83:dbl[unit], error out=w84:errorcluster)
      n18 = Variant To Data(error in=w113, type=T4[] [] ("Stored ROIs in"), Variant=w114) -> (data=w93:T4[], error out=w109:errorcluster)
      n19 = node(w83) -> (w82:dbl)
      n20 = Bundle By Name(cluster=cluster{"Image Sum":T2, "Image Array":T2[]} {"Image Sum"=refnum, "Image Array"=[]} ("Images"), "Image Sum"=w64, "Image Array"=w63) -> (w104:cluster{"Image Sum":T2, "Image Array":T2[]})
      n21 = call "AlliGator Get Sum Image Threshold.vi"("error in (no error)"=w110, "Pixel Counts Constraints"=w111, "Image in"=w64) -> ("error out"=w75:errorcluster, "Pixel Threshold Low"=w107:sgl, "Pixel Threshold High"=w108:sgl, "Y Resolution"=w44:i32, "X Resolution"=w45:i32)  [unwired: 2 in, 2 out]
      n22 = Array Size(array=w93) -> (size(s)=w43:i32)
      n23 = Multiply(x=w45, y=w44) -> (x*y=w42:i32)
      n24 = Equal?(x=w42, y=w43) -> (x = y?=w39:bool)
      n25 = Merge Errors(w75, w109, w106, w84, w99) -> (w66:errorcluster)
      n26 = case shown="1, Default" w43 {
        selector: w43 -> [_ w168]
        tunnel: w108 -> [_ w213]
        tunnel: w107 -> [_ w212]
        tunnel: w105 -> [_ w211]
        tunnel: w104 -> [_ w210]
        tunnel: w63 -> [_ w209]
        tunnel: w103 -> [_ w159]
        tunnel: [_ w206] -> w102
        tunnel: [_ w203] -> w98
        tunnel: w93 -> [_ w202]
        tunnel: w92 -> [_ w201]
        tunnel: [w130 w200] -> w89
        tunnel: w82 -> [_ w198]
        tunnel: w81 -> [w131 w196]
        tunnel: [w131 w194] -> w80
        tunnel: [_ w138] -> w79
        tunnel: [w132 w193] -> w78
        tunnel: w77 -> [_ w177]
        tunnel: w76 -> [w132 w175]
        tunnel: w66 -> [_ w187]
        tunnel: w74 -> [_ w181]
        tunnel: [w129 w180] -> w73
        tunnel: w72 -> [w129 w164]
        tunnel: [w128 w178] -> w69
        tunnel: w68 -> [w128 w165]
        tunnel: w67 -> [_ w171]
        tunnel: w49 -> [w126 w162]
        tunnel: w48 -> [w125 w163]
        tunnel: [w126 w158] -> w47
        tunnel: [w125 w160] -> w46
        tunnel: w41 -> [w124 w146]
        tunnel: [w124 w152] -> w40
        tunnel: w39 -> [_ w145]
        tunnel: w38 -> [w123 w144]
        tunnel: w37 -> [w122 w148]
        tunnel: [w123 w151] -> w36
        tunnel: [w122 w150] -> w35
        tunnel: [w121 w142] -> w34
        tunnel: w33 -> [w121 w141]
        tunnel: w32 -> [w120 w140]
        tunnel: [w120 w139] -> w31
        frame 0 {
          n27 = One Button Dialog(message="All ROIs Decay Fit: no ROI defined!") -> ()  [unwired: 1 in, 1 out]
          n28 = call "Play Error Sound.vi"() -> ()  [unwired: 27 in, 1 out]
          n29 = xnode "Error Ring"() -> ("error out"=w130:errorcluster)
        }
        frame 1, Default {
          # "the second pass idea requires another way to pass best fit parameters to // loops: now inactive"
          # "invalid fit [idx]\noriginally: all"
          n30 = call "AlliGator Get-Set Decay Preprocessing Parameters.vi"("Get (F)/Set"=FALSE, "Error In"=w187) -> ("Error Out"=w157:errorcluster, "Decay Preprocessing Parameters out"=w161:T38)  [unwired: 8 in]
          n31 = call "AlliGator Get Fit Options & Parameters.vi"("error in (no error)"=w157, "Reset Fit Options & Parameters"=TRUE) -> ("error out"=w156:errorcluster, "Use Legacy Fitting Approach"=w155:bool, "Decay Fit Options & Parameters"=w153:T27)  [unwired: 7 in]
          n32 = call "AlliGator New NLSF Parameter Map Resolution.vi"("Is Full Image Parameter Map"=w145, "Old NLSF Parameters Map Y Resolution"=w148, "Old NLSF Parameters Map X Resolution"=w144) -> (2:"New NLSF Parameters Map X Resolution"=w147:i32, 3:"New NLSF Parameters Map X Resolution"=w149:i32)  [unwired: 7 in]
          n33 = Array Size(array=w209) -> (size(s)=w208:i32)
          n34 = call "AlliGator Get IRF Values & Locations.vi"("[IRF Data]"=w177) -> ("IRF Locations"=w174:cluster{"X":i32, "Y":i32}[], "[IRF Values]"=w176:dbl[][])  [unwired: 9 in]
          n35 = call "Embedded Progress Bar Q.vi"("Progress Bar Queue Name"="AlliGator Progress Bar Q") -> ("Progress Bar Queue"=w170:refnum<queue>)  [unwired: 6 in]
          n36 = call "Linear Ramp [I32].vi"("# Elements"=w168) -> ("Ramp"=w186:i32[])  [unwired: 8 in]
          n37 = call "AlliGator Get Decay Time Axis v2.vi"("Number of Gates"=w208) -> ("t Array"=w207:dbl[unit][])  [unwired: 14 in]
          n38 = call "Send Embedded Progress Bar Update.vi"("Max Iterations N"=w168, "Current Iteration i (i or -1: standard or || iteration; 0 or -2: first standard or || iteration)"=-2 ("Current Iteration i (i or -1: standard or || iteration; 0 or -2: first standard or || iteration)"), "Progress Bar Queue in"=w170) -> ("Error Out"=w166:errorcluster, "Progress Bar Queue out"=w169:refnum<queue>)  [unwired: 7 in]
          n39 = node(w207) -> (w205:dbl[])
          n40 = for {
            N: 1 -> [_]
            tunnel: w213 -> [w265]
            tunnel: w212 -> [w264]
            tunnel: w211 -> [w263]
            tunnel: w210 -> [w262]
            tunnel: w159 -> [w261]
            tunnel: [w221] -> w206 mode=concatenating
            tunnel: w205 -> [w260]
            tunnel: "Abort Fit" ("Abort Button Name (Abort)") -> [w259]
            tunnel: [w258] -> w203
            tunnel: w201 -> [w256]
            tunnel: w172 -> [w253]
            tunnel: [w251] -> w199 mode=concatenating
            tunnel: w198 -> [w250]
            shift-right: [w245] -> w138
            shift-left: _ -> [w248]
            tunnel: w181 -> [w254]
            tunnel: [FALSE ("Abort?")] -> w197
            shift-right: [w246] -> _
            shift-left: dbl[][] [] -> [w236]
            tunnel: [w249] -> w195 mode=concatenating
            tunnel: [w243] -> w191
            tunnel: w156 -> [w241]
            tunnel: w176 -> [w255]
            shift-right: [w240] -> _
            shift-left: i32[] [] -> [w235]
            tunnel: w202 -> [w257]
            tunnel: w168 -> [w252]
            shift-right: [w239] -> _
            shift-left: w186 -> [w227]
            tunnel: [w234] -> w179 mode=concatenating
            tunnel: w174 -> [w233]
            tunnel: w161 -> [w232]
            tunnel: w171 -> [w228]
            tunnel: w169 -> [w237]
            tunnel: [w242] -> w190
            tunnel: w166 -> [w225]
            tunnel: w153 -> [w224]
            tunnel: w155 -> [w223]
            tunnel: [w218] -> w143
            tunnel: [w217] -> w137
            i -> [w231]
            stop <- w244 stop-if-true
            # "invalid fit idx\n(unused)"
            # "First Loop: try all decays, Second Loop: try all the failed decay fit again with parameters from nearby successful fits"
            n41 = Array Size(array=w227) -> (size(s)=w226:i32)
            n42 = for {
              tunnel: w257 -> [w293] mode=indexing
              tunnel: w265 -> [w313]
              tunnel: w264 -> [w312]
              tunnel: w262 -> [w311]
              tunnel: w263 -> [w310]
              tunnel: w260 -> [w309]
              tunnel: w261 -> [w308]
              tunnel: [w307] -> w221 mode=indexing if=w301
              tunnel: w241 -> [w291]
              tunnel: w259 -> [w306]
              tunnel: [w305] -> w251 mode=indexing if=w273
              tunnel: [w304] -> w258 mode=indexing if=w273
              tunnel: w254 -> [w302]
              tunnel: [w303] -> w249 mode=indexing if=w273
              tunnel: w252 -> [w288]
              tunnel: w256 -> [w300]
              tunnel: w255 -> [w292]
              tunnel: [w277] -> w245
              tunnel: w253 -> [w299]
              tunnel: [w297] -> w243
              tunnel: w250 -> [w295]
              tunnel: w248 -> [w294]
              tunnel: [w285] -> w239 mode=indexing if=w287
              tunnel: w227 -> [w290]
              tunnel: [w282] -> w234 mode=indexing if=w273
              tunnel: w233 -> [w281]
              tunnel: w232 -> [w280]
              tunnel: w237 -> [w298]
              tunnel: [w296] -> w242
              tunnel: w225 -> [w279]
              tunnel: w236 -> [w283]
              tunnel: [w286] -> w246 mode=indexing if=w273
              tunnel: w235 -> [w284]
              tunnel: [w285] -> w240 mode=indexing if=w273
              tunnel: w224 -> [w276]
              tunnel: w223 -> [w275]
              tunnel: [w274] -> w222 mode=indexing if=w273
              tunnel: [w272] -> w217
              i -> [w289]
              n43 = global read "AlliGator Abort.vi" "Abort?"() -> (w277:bool)
              n44 = case shown="False" w277 {
                selector: w277 -> [w318 _]
                tunnel: w313 -> [w350 _]
                tunnel: w312 -> [w349 _]
                tunnel: w311 -> [w348 _]
                tunnel: w310 -> [w347 _]
                tunnel: w309 -> [w346 _]
                tunnel: w308 -> [w345 _]
                tunnel: [w344 _] -> w307
                tunnel: w306 -> [w343 _]
                tunnel: [w342 w440] -> w305
                tunnel: [w341 _] -> w304
                tunnel: [w340 _] -> w303
                tunnel: w302 -> [w339 _]
                tunnel: [w338 _] -> w301
                tunnel: w300 -> [w337 _]
                tunnel: w299 -> [w336 _]
                tunnel: w295 -> [w335 _]
                tunnel: w294 -> [_ _]
                tunnel: w293 -> [w334 _]
                tunnel: w292 -> [w333 _]
                tunnel: w291 -> [w332 w440]
                tunnel: w290 -> [w331 _]
                tunnel: w289 -> [w329 _]
                tunnel: w288 -> [w328 _]
                tunnel: [w327 _] -> w287
                tunnel: [w326 _] -> w286
                tunnel: [w325 _] -> w285
                tunnel: w284 -> [w324 _]
                tunnel: w283 -> [w323 _]
                tunnel: [w322 _] -> w282
                tunnel: w281 -> [w321 _]
                tunnel: w280 -> [w320 _]
                tunnel: [w319 _] -> w273
                tunnel: w276 -> [w317 _]
                tunnel: w275 -> [w316 _]
                tunnel: [w315 _] -> w274
                tunnel: [w314 _] -> w272
                frame False {
                  n45 = Search 1D Array(1D array=w331, element=w329) -> (index of element=w330:i32)  [unwired: 1 in]
                  n46 = case shown="0, Default" w330 {
                    tunnel: w350 -> [w396 _]
                    tunnel: w349 -> [w395 _]
                    tunnel: w348 -> [w394 _]
                    tunnel: w347 -> [w393 _]
                    tunnel: w346 -> [w391 _]
                    tunnel: w345 -> [w387 _]
                    tunnel: [w386 _] -> w344
                    tunnel: w343 -> [w385 _]
                    tunnel: [w384 _] -> w342
                    tunnel: [w383 _] -> w341
                    tunnel: [w382 _] -> w340
                    tunnel: w339 -> [w381 _]
                    tunnel: [w380 _] -> w338
                    tunnel: w337 -> [w379 _]
                    tunnel: w336 -> [w375 _]
                    tunnel: w328 -> [w374 _]
                    tunnel: w335 -> [w373 _]
                    tunnel: w334 -> [w372 _]
                    tunnel: w333 -> [w362 _]
                    tunnel: [w371 _] -> w326
                    tunnel: w329 -> [w351 _]
                    tunnel: w332 -> [w367 _]
                    tunnel: [w370 _] -> w325
                    tunnel: [w368 _] -> w319
                    tunnel: [w369 _] -> w327
                    tunnel: w324 -> [_ _]
                    tunnel: w323 -> [_ _]
                    tunnel: w329 -> [_ _]
                    tunnel: [w365 _] -> w322
                    tunnel: w321 -> [w364 _]
                    tunnel: w320 -> [w359 _]
                    tunnel: w318 -> [w358 _]
                    tunnel: w317 -> [w356 _]
                    tunnel: w316 -> [w355 _]
                    tunnel: [w353 _] -> w315
                    tunnel: [w352 _] -> w314
                    frame 0, Default {
                      # "same location?"
                      # "Note: the following is no longer applicable [no good fit: try again (or for the first time)]"
                      n47 = Unbundle By Name(w372) -> ("ROI Descriptor"=w392:T5, "ROI Name"=w386:string)
                      n48 = call "AlliGator Compute ROI Decay.vi"("Pixel Threshold High"=w396, "Loop ID"=w351, "Pixel Threshold Low"=w395, "error in (no error)"=w367, "Decay Peak  Constraints"=w393, "ROI Descriptor"=w392, "Images"=w394) -> ("error out"=w366:errorcluster, "# Valid Pixels"=w388:i32, "ROI Center"=w363:cluster{"X":i32, "Y":i32}, "Decay Points"=w390:dbl[], "# Pixels"=w354:i32)
                      n49 = To Double Precision Float(number=w363) -> (double precision float=w378:cluster{"X":dbl, "Y":dbl})
                      n50 = Search 1D Array(1D array=w364, element=w363) -> (index of element=w360:i32)  [unwired: 1 in]
                      n51 = Cluster To Array(cluster=w378) -> (array=w377:dbl[])
                      n52 = Index Array(array=w362, index (row)=w360) -> (element=w361:dbl[])  [unwired: 1 in]
                      n53 = Greater Or Equal To 0?(x=w360) -> (x >= 0?=w357:bool)
                      n54 = Bundle(w391, "Decay Points"=w390) -> (w389:cluster{dbl[], "Decay Points":dbl[]})  [unwired: 1 in]
                      n55 = Compound Arithmetic op=AND(w357, invert w358) -> (w376:bool)
                      n56 = case shown="True" w376 {
                        tunnel: w389 -> [_ w436]
                        tunnel: w388 -> [_ w435]
                        tunnel: w387 -> [_ w434]
                        tunnel: w386 -> [_ w431]
                        tunnel: w385 -> [_ _]
                        tunnel: [w397 w415] -> w384
                        tunnel: [_ w429] -> w383
                        tunnel: [_ w418] -> w382
                        tunnel: w381 -> [_ w427]
                        tunnel: w374 -> [_ w426]
                        tunnel: w351 -> [_ w411]
                        tunnel: [_ w425] -> w380
                        tunnel: w379 -> [_ w423]
                        tunnel: w377 -> [_ w400]
                        tunnel: w366 -> [w397 w421]
                        tunnel: w375 -> [_ w409]
                        tunnel: w373 -> [_ w408]
                        tunnel: [_ w416] -> w371
                        tunnel: [_ w411] -> w370
                        tunnel: [_ TRUE] -> w368
                        tunnel: [_ w406] -> w365
                        tunnel: w361 -> [_ w405]
                        tunnel: w359 -> [_ w404]
                        tunnel: w356 -> [_ w399]
                        tunnel: w355 -> [_ w403]
                        tunnel: w354 -> [_ w401]
                        tunnel: [_ w401] -> w353
                        tunnel: [_ w398] -> w352
                        frame False {
                          # "Not the same ROI coordinates"
                        }
                        frame True {
                          w432 = T45 {"Multiplot XY Graph"=refnum, "Mouse Coordinates"={"Horizontal"=0, "Vertical"=0}, "Plot Index"=-1, "Flag"=FALSE}  # Flag: non-interactive
                          n57 = call "AlliGator Preprocess Decay v3.vi"("Decay Preprocessing Parameters"=w404, "Error In"=w421, "Time-Gated Reference Decay"=w434, "# Pixels"=w435, "Decay (in)"=w436) -> ("Error Out"=w417:errorcluster, "Decay (out)"=w433:T48)  [unwired: 3 in, 2 out]
                          n58 = Bundle("IRF Array Time Axis"=w423, "[IRF Values]"=w405) -> (w422:T49)  [unwired: 1 in]
                          n59 = call "AlliGator Fit Decay.vi"("Selected Plot Info + Flag"=w432, "Decay Fit Options & Parameters"=w399, "Current Decay Name"=w431, "Current Decay"=w433, "Reference Decay"=w422, "error in (no error)"=w417, "Use Legacy Fitting Approach"=w403) -> ("Best Fit Parameters (All)"=w416:dbl[], "Delta Best Fit Parameters (All)"=w410:dbl[], "R^2"=w402:dbl, "Reduced Chi^2"=w430:dbl, "Error Out"=w415:errorcluster)  [unwired: 4 out]
                          n60 = Unbundle By Name(w399) -> ("Fit Options.Fit Model"=w398:T29)
                          n61 = Unbundle By Name(w415) -> ("status"=w414:bool)
                          n62 = call "Keep String in Array.vi"("Current Index"=w411, "Number of Elements"=w426) -> ("Keep String"=w424:bool)  [unwired: 9 in]
                          n63 = Build Array (concatenate)(w416, w402, w430) -> (w420:dbl[])
                          n64 = Not(x=w414) -> (.not. x?=w413:bool)
                          n65 = call "Get Decay Fit Parameters.vi"("Laser Period"=w408, "Decay Fit Output Options"=w409, "Decay Fit Parameters"=w420) -> ("Displayed Decay Fits Parameters"=w419:dbl[])  [unwired: 7 in, 1 out]
                          n66 = Build Array (concatenate)(w400, w420) -> (w428:dbl[])
                          n67 = call "Get Decay Fit Parameters.vi"("Laser Period"=w408, "Decay Fit Output Options"=w409, "Decay Fit Parameters"=w410) -> ("Displayed Decay Fits Parameters"=w407:dbl[])  [unwired: 7 in, 1 out]
                          n68 = case shown="True" w427 {
                            tunnel: [_ w439] -> w429
                            tunnel: w428 -> [_ w438]
                            frame False {
                            }
                            frame True {
                              n69 = Array To Spreadsheet String(array=w438, 3:"%#g" ("format string")) -> (spreadsheet string=w439:string)  [unwired: 1 in]
                            }
                          }
                          n70 = Build Array (concatenate)(w400, w419) -> (w418:dbl[])
                          n71 = Build Array (concatenate)(w400, w407) -> (w406:dbl[])
                          n72 = Compound Arithmetic op=AND(w424, w413) -> (w425:bool)
                        }
                      }
                      n73 = Not(x=w368) -> (.not. x?=w369:bool)
                    }
                    frame -1 {
                      # "already successful: do nothing"
                    }
                  }
                }
                frame True {
                }
              }
              n74 = call "Send Embedded Progress Bar Update.vi"("Error In"=w279, "Current Iteration i (i or -1: standard or || iteration; 0 or -2: first standard or || iteration)"=-1 ("Current Iteration i (i or -1: standard or || iteration; 0 or -2: first standard or || iteration)"), "Progress Bar Queue in"=w298) -> ("Error Out"=w297:errorcluster, "Progress Bar Queue out"=w296:refnum<queue>)  [unwired: 7 in]
            }
            n75 = case shown="0, Default" w231 {
              tunnel: [w267 w271] -> w229
              tunnel: w226 -> [_ w269]
              frame 0, Default {
                n76 = call "Current Date & Time String (High Precision).vi"() -> ("on <Date> at <Time>"=w266:string)  [unwired: 8 in, 3 out]
                n77 = Format Into String(format string="All ROIs Non-Interactive Decay Fit (Individual IRFs) started %s", w266) -> (resulting string=w267:string)  [unwired: 2 in, 1 out]
              }
              frame 1 {
                n78 = Format Into String(format string="Re-processing %d decays...", w269) -> (resulting string=w271:string)  [unwired: 2 in, 1 out]
              }
            }
            n79 = call "Message Style.vi"() -> ("Message Formatting"=w230:T50)
            n80 = call "Send Message to Notebook.vi"("Text Formatting"=w230, "Message"=w229, "Notebook Queue"=w228) -> ()  [unwired: 5 in, 2 out]
            n81 = Empty Array?(array=w239) -> (empty?=w238:bool)
            n82 = Add Array Elements(numeric array=w222) -> (sum=w219:i32)
            n83 = Array Size(array=w221) -> (size(s)=w220:i32)
            n84 = Equal?(x=w220, y=w219) -> (x = y?=w218:bool)
            n85 = Compound Arithmetic op=OR(w238, w245) -> (w244:bool)
          }
          n86 = flat-sequence {
            tunnel: [w215] -> w182
            tunnel: [w214] -> w172
            frame #0 {
              n87 = call "AlliGator Get Fit Output Options.vi"("All Parameters?"=TRUE) -> ("Decay Fit Output Options"=w214:T52)  [unwired: 8 in, 2 out]
              n88 = Unbundle By Name(w214) -> ("Decay Fit Parameter Array"=w215:T39[])
            }
          }
          n89 = global write "AlliGator Abort.vi" "Abort?"(w197) -> ()
          n90 = call "Send Embedded Progress Bar Update.vi"("Stop Progress Bar (F)"=TRUE ("Hide Progress Bar"), "Error In"=w191, "Progress Bar Queue in"=w190) -> ("Error Out"=w189:errorcluster)  [unwired: 7 in, 1 out]
          n91 = Select(t=w162, s=w138, f=w159) -> (s? t:f=w158:cluster{"t Array":dbl[], "I Array":dbl[]})
          n92 = Select(t=w165, s=w138, f=w179) -> (s? t:f=w178:dbl[][])
          n93 = Select(t=w196, s=w138, f=w195) -> (s? t:f=w194:dbl[][])
          n94 = Select(t=w175, s=w138, f=w182) -> (s? t:f=w193:T39[])
          n95 = Select(t=w163, s=w138, f=w161) -> (s? t:f=w160:T38)
          n96 = Merge Errors(w199, w189) -> (w200:errorcluster)
          n97 = Select(t=w146, s=w138, f=w145) -> (s? t:f=w152:bool)
          n98 = Select(t=w164, s=w138, f=w153) -> (s? t:f=w180:T27)
          n99 = Select(t=w148, s=w138, f=w147) -> (s? t:f=w150:i32)
          n100 = Select(t=w141, s=w138, f=w143) -> (s? t:f=w142:bool)
          n101 = Select(t=w144, s=w138, f=w149) -> (s? t:f=w151:i32)
          n102 = Select(t=w140, s=w138, f=w137) -> (s? t:f=w139:T29)
        }
      }
      n103 = call "AlliGator Get Tabulated Results Header (Decay Fit).vi"() -> ("Tabulated Results Header"=w97:string)  [unwired: 10 in, 1 out]
      n104 = call <vilib>:"Clear Errors.vi"("error in (no error)"=w89, "specific error code to clear (0: all)"=w70) -> ("error out"=w71:errorcluster)  [unwired: 4 in, 1 out]
      n105 = Build Array (concatenate)(w97, w98) -> (w96:string[])
      n106 = in-place-cluster #2("Fit Model"=w31, "NLSF Parameters Map X Resolution"=w36, "NLSF Parameters Map Y Resolution"=w35, "Is Full Image Parameters Map"=w40, "Fit Options: Decay Preprocessing Parameters"=w46, "Fit Options: Reference Decay"=w47, "Current Dataset Images 1.SGL Image Sum"=w62, "Current Dataset Images 1.SGL Gate Images"=w61, "Current Dataset Images 2.SGL Image Sum"=w60, "Current Dataset Images 2.SGL Gate Images"=w59, "Reference Decay"=w103, "[[Multiple Decays Fit Parameters]]"=w80, "IRF Array Time Axis"=w92, "[[IRFs]]"=w77, "[Decay Fit Parameter Names]"=w78, "Decay Fit Options & Parameters"=w73, "[[Multiple Decays Fit Parameter SDVs]]"=w69, "Is Single-Pixels Parameters Map"=w34) -> (w29:T6)
      n107 = case shown="False" w79 {
        tunnel: w96 -> [w447 _]
        tunnel: [w446 w460] -> w95
        tunnel: w71 -> [w445 w460]
        tunnel: "Choose or enter file path for tabulated fits results:" ("prompt (Choose or enter file path)") -> [w444 _]
        tunnel: "Fit Results saved in %s" ("format string") -> [w443 _]
        tunnel: [w442 "All ROIs Decay Fit (Non-interacitve, Individual IRF) aborted by user."] -> w90
        tunnel: w74 -> [w441 _]
        frame False {
          # "Don't Abort"
          n108 = case shown="True" w441 {
            tunnel: w447 -> [_ w458]
            tunnel: [w448 w451] -> w446
            tunnel: w445 -> [w448 w457]
            tunnel: w444 -> [_ w456]
            tunnel: w443 -> [_ w450]
            tunnel: [_ w449] -> w442
            frame False {
            }
            frame True {
              n109 = Write to Text File(prompt (Choose or enter file path)=w456, text=w458, error in=w457) -> (refnum out=w455:refnum<file>, error out=w454:errorcluster)  [unwired: 1 in, 1 out]
              n110 = Close File(refnum=w455, error in=w454) -> (path=w452:path, error out=w453:errorcluster)
              n111 = Format Into String(format string=w450, error in=w453, w452) -> (resulting string=w449:string, error out=w451:errorcluster)  [unwired: 1 in]
            }
          }
        }
        frame True {
          # "Abort"
        }
      }
    }
    n112 = in-place-dvr #1(w29) -> (→"AlliGator Internal Variables DVR":refnum<data-value>)  [unwired: 1 out]
  }
  n113 = call "High Resolution Timing.vi"("relative seconds (NaN)"=w14, "Error In"=w9) -> ("elapsed (relative) seconds"=w13:dbl, "Error Out"=w7:errorcluster)  [unwired: 15 in, 1 out]
  n114 = call "Concatenate String Array.vi"("Max Number of Elements (None: -1)"=8 ("Max Number of Elements (None: 1)"), "Separator (TAB)"=", ", "String Array"=w11) -> ("Formatted String"=w12:string)  [unwired: 8 in]
  n115 = call "Current Date & Time String (High Precision).vi"("Error In"=w7) -> ("Error Out"=w6:errorcluster, "on <Date> at <Time>"=w1:string)  [unwired: 7 in, 2 out]
  n116 = Format Into String(format string="All ROIs Decay Fit (%d):\n%s completed on %s\nCPU: %#g s\n%s", error in=w6, w5, w12, w1, w13, w8) -> (resulting string=→"Message":string, error out=→"error out":errorcluster)  [unwired: 1 in]
